vi "setFinishDirectOrKickoff.vi"(8 "error in (no error)":errorcluster, 10 "Game":refnum<class "Game.lvclass">, 11 "Play in":refnum<class "Play.lvclass">) -> (0 "error out":errorcluster, 2 "Game out":refnum<class "Game.lvclass">, 3 "Play out":refnum<class "Play.lvclass">)   [LabVIEW 2020, in "Play.lvclass"]
uses:
  Play.lvclass
  Game_class/Game.lvclass
  Referee_class/command_interpreted.ctl
  Game_class/Game.lvclass/Game.ctl
  Ally_class/Ally.lvclass/Ally.ctl
  Events_class/Events.lvclass/Events.ctl
  Referee_class/Referee.lvclass/Referee.ctl
  Ball_class/Ball.lvclass/Ball.ctl
  Ally_class/Write DirectOrKickoff.vi
  Game_class/Read OffensiveTeam.vi
  Game_class/Read BallRef.vi
  Game_class/Read EventsRef.vi
  Game_class/Read Referee.vi
  Referee_class/Read command_interpreted.vi
  Events_class/Read kick.vi
  Ball_class/Read velocityNorm.vi
  Ally_class/Read DirectOrKickoff.vi
  Game_class/Write OffensiveTeam.vi
  <vilib>/Analysis/_algsub.llb/Vector Norm.vi
  <vilib>/Analysis/_algsub.llb/Real Vector Norm.vi
  Ally_class/Ally.lvclass
  Ball_class/Ball.lvclass
  Events_class/Events.lvclass
  Referee_class/Referee.lvclass
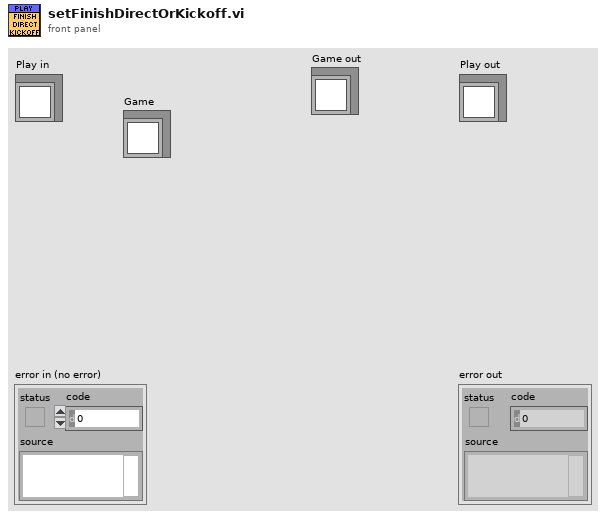
[diagram p1: front panel]
types:
  T1 = typedef "command_interpreted.ctl" = enum16{"Goal Ally", "Goal Enemy", "Ball Placement Enemy", "Ball Placement Ally", "Normal Half Time", "Extra Time  Break", "Extra Half Time", "None", "Post Game", "PKA Normal Start", "Prepare Kickoff Ally", "PKE Normal Start", "Prepare Kickoff Enemy", "Force Start", "Halt", "Timeout", "Prepare Penalty Ally", "Prepare Penalty Enemy", "PPA NormalStart", "PPE Normal Start", "Indirect Free Ally", "Direct Free Enemy", "Direct Free Ally", "Indirect Free Enemy", "Stop"}
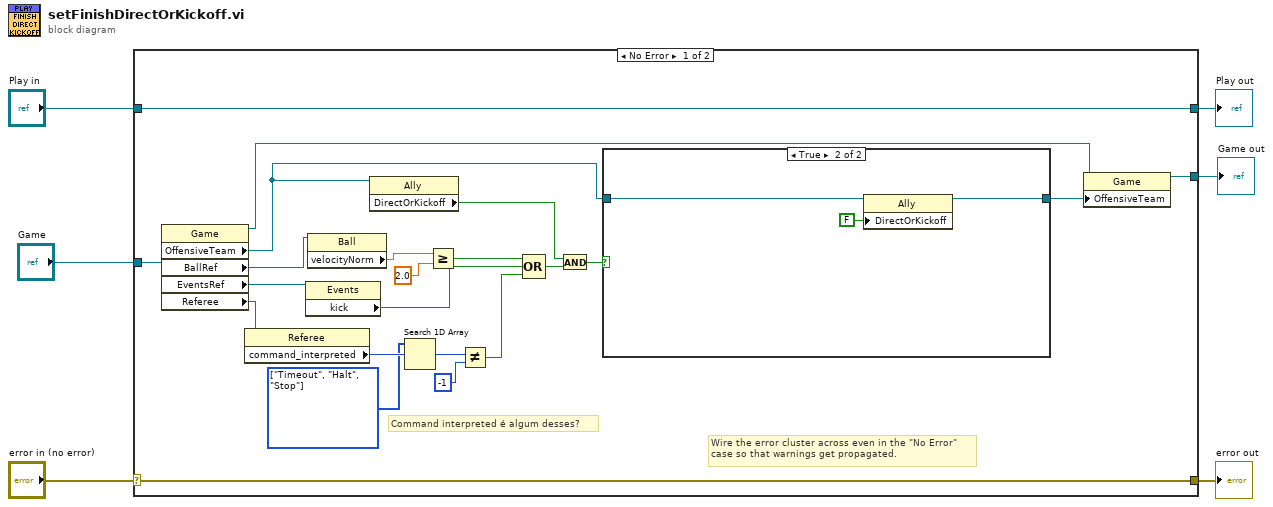
[diagram p0: block diagram]
diagram:
  n1 = case shown="No Error" "error in (no error)" {
    selector: "error in (no error)" -> [w27 w34]
    tunnel: [w27 w34] -> w5
    tunnel: [w28 w33] -> w3
    tunnel: "Play in" -> [w28 w33]
    tunnel: "Game" -> [w26 _]
    tunnel: [w13 _] -> w1
    frame No Error {
      w10 = T1[] [enum."Timeout", enum."Halt", enum."Stop"] items=["Goal Ally", "Goal Enemy", "Ball Placement Enemy", "Ball Placement Ally", "Normal Half Time", "Extra Time  Break", "Extra Half Time", "None", "Post Game", "PKA Normal Start", "Prepare Kickoff Ally", "PKE Normal Start", "Prepare Kickoff Enemy", "Force Start", "Halt", "Timeout", "Prepare Penalty Ally", "Prepare Penalty Enemy", "PPA NormalStart", "PPE Normal Start", "Indirect Free Ally", "Direct Free Enemy", "Direct Free Ally", "Indirect Free Enemy", "Stop"] ("1D array")
      # "Command interpreted é algum desses?"
      # "Wire the error cluster across even in the \"No Error\"\ncase so that warnings get propagated."
      n2 = property class="Game"(reference=w26) -> (reference out=w15:refnum<class "Game.lvclass">, "OffensiveTeam"=w16:refnum<class "Ally.lvclass">, "BallRef"=w23:refnum<class "Ball.lvclass">, "EventsRef"=w25:refnum<class "Events.lvclass">, "Referee"=w12:refnum<class "Referee.lvclass">)  [unwired: 1 in, 1 out]
      n3 = property class="Referee"(reference=w12) -> ("command_interpreted"=w11:T1)  [unwired: 1 in, 2 out]
      n4 = property class="Events"(reference=w25) -> ("kick"=w24:bool)  [unwired: 1 in, 2 out]
      n5 = property class="Ball"(reference=w23) -> ("velocityNorm"=w22:dbl)  [unwired: 1 in, 2 out]
      n6 = property class="Ally"(reference=w16) -> ("DirectOrKickoff"=w17:bool)  [unwired: 1 in, 2 out]
      n7 = Search 1D Array(1D array=w10, element=w11) -> (index of element=w9:i32)  [unwired: 1 in]
      n8 = Greater Or Equal?(x=w22, y=2.0) -> (x >= y?=w20:bool)
      n9 = Not Equal?(x=w9, y=-1) -> (x != y?=w7:bool)
      n10 = Compound Arithmetic op=OR(w20, w24, w7) -> (w19:bool)
      n11 = And(x=w17, y=w19) -> (x .and. y?=w18:bool)
      n12 = case shown="True" w18 {
        tunnel: w16 -> [w29 w32]
        tunnel: [w29 w30] -> w14
        frame False {
        }
        frame True {
          n13 = property class="Ally"(reference=w32, "DirectOrKickoff"=FALSE) -> (reference out=w30:refnum<class "Ally.lvclass">)  [unwired: 1 in, 1 out]
        }
      }
      n14 = property class="Game"(reference=w15, "OffensiveTeam"=w14) -> (reference out=w13:refnum<class "Game.lvclass">)  [unwired: 1 in, 1 out]
    }
    frame Error {
    }
  }
  "error out" <- w5
  "Play out" <- w3
  "Game out" <- w1
